vi "configureTrigger.vi"(0 "HGF_IMAQDevice":refnum<class "HGF_IMAQDevice.lvclass">, 1 "Type":u32(ring) items=["External"=0, "RTSI"=1, "ISO In"=2, "Scaled Encoder"=5, "Software Trigger"=6], 2 "Line Number (0)":u32, 3 "Frame timeout (ms)":u32=1000, 4 "Action":u32(ring) items=["Disabled", "Trigger start of acquisition", "Trigger start of each buffer list", "Trigger each buffer", "Trigger each line (linescan)", "Trigger end of acquisition"], 5 "error in (no error)":errorcluster, 6 "Activation":u32(ring) items=["Rising Edge", "Falling Edge", "AnyEdge", "LevelHigh", "LevelLow"], 7 "Delay (0ms)":cluster{"Value":dbl, "Units":u32}={"Value"=0.0, "Units"=5} {"Units" items=["Scaled Encoder Counts"=4, "Milliseconds"=5]}, 8 "Mode (off)":T1(ring), 9 "Skip trigger (linescan only) (0)":u32) -> (14 "dup HGF_IMAQDevice":refnum<class "HGF_IMAQDevice.lvclass">, 19 "error out":errorcluster)   [LabVIEW 2014, in "HGF_IMAQ.lvlib" / "HGF_IMAQDevice.lvclass"]
doc: "Configures the trigger conditions for an acquisition. Use this VI before any acquisition VI to setup a triggered image acquisition."
uses:
  HGF_IMAQDevice.lvclass
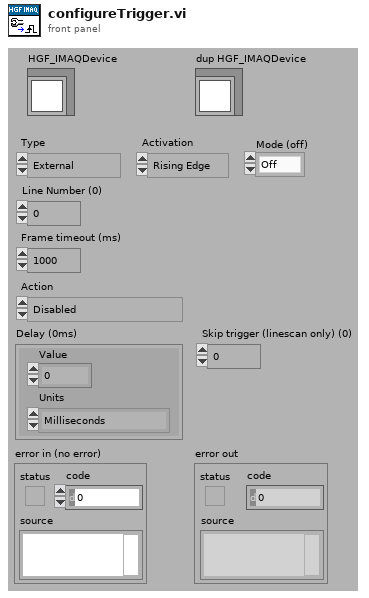
[diagram p1: front panel]
types:
  T1 = enum16{"Off", "Mode 0", "Mode 1", "Mode 2", "Mode 3", "Mode 4", "Mode 5"}
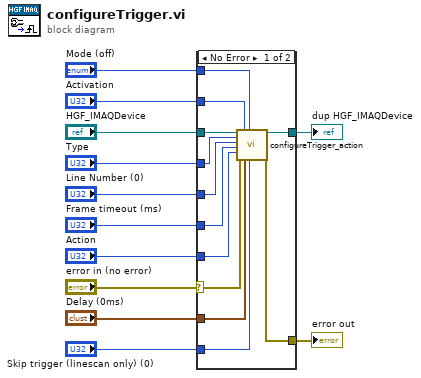
[diagram p0: block diagram]
diagram:
  n1 = case shown="No Error" "error in (no error)" {
    selector: "error in (no error)" -> [w22 w26]
    tunnel: [w21 w26] -> w11
    tunnel: [w23 w25] -> w9
    tunnel: "HGF_IMAQDevice" -> [w24 w25]
    tunnel: "Activation" -> [w20 _]
    tunnel: "Type" -> [w19 _]
    tunnel: "Line Number (0)" -> [w18 _]
    tunnel: "Frame timeout (ms)" -> [w17 _]
    tunnel: "Action" -> [w16 _]
    tunnel: "Delay (0ms)" -> [w15 _]
    tunnel: "Skip trigger (linescan only) (0)" -> [w14 _]
    tunnel: "Mode (off)" -> [w13 _]
    frame No Error {
      n2 = call-dynamic "configureTrigger_action.vi"("HGF_IMAQDevice"=w24, "Type"=w19, "Line Number"=w18, "Frame timeout (ms)"=w17, "Action"=w16, "error in (no error)"=w22, "Activation"=w20, "Delay"=w15, "Mode"=w13, "Skip trigger (linescan only)"=w14) -> ("dup HGF_IMAQDevice"=w23:refnum<class "HGF_IMAQDevice.lvclass">, "error out"=w21:errorcluster)  [unwired: 8 in]
    }
    frame Error {
    }
  }
  "error out" <- w11
  "dup HGF_IMAQDevice" <- w9
